vi "HandleError.vi"(8 "ErrorArray":errorcluster[](array[cluster])) -> (0 "ErrorArray":errorcluster[](array[cluster]), 4 "Stop":bool)   [LabVIEW 2014, in "TestBase.lvclass"]
uses:
  TestBase.lvclass
  Queue/clQueMsgType.ctl
  <vilib>/Utility/error.llb/Error Cluster From Error Code.vi
  <vilib>/ErrorRing/Error Ring.xnode
  <userlib>/NIST/NISTErrorLib/NISTErrorLib.lvlib
panel:
  out "XML_Out":string[](array[string])
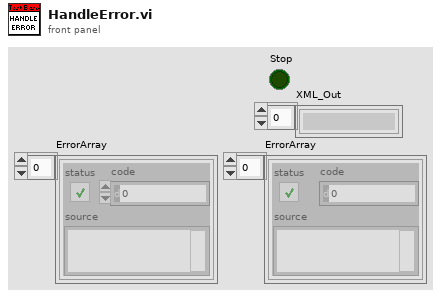
[diagram p1: front panel]
types:
  T1 = typedef "TestBase.lvclass/clQueMsgType.ctl" = cluster{"Message":string, "Data":variant}
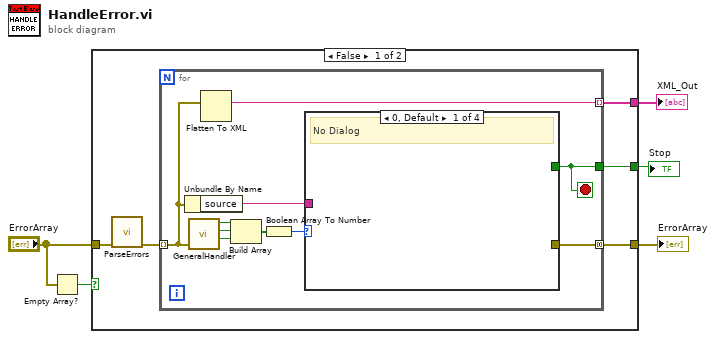
[diagram p0: block diagram]
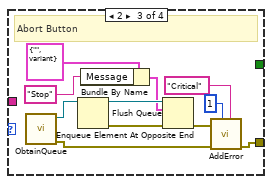
[diagram p4: hidden frame]
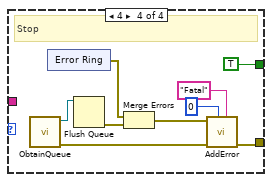
[diagram p5: hidden frame]
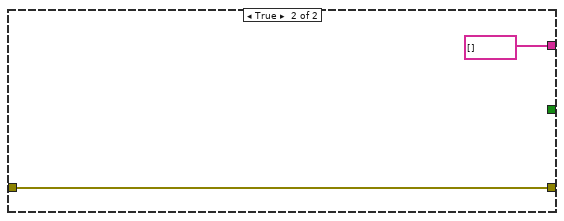
[diagram p6: hidden frame]
diagram:
  n1 = Empty Array?(array="ErrorArray") -> (empty?=w5:bool)
  n2 = case shown="False" w5 {
    tunnel: "ErrorArray" -> [w10 w48]
    tunnel: [w7 w48] -> w3
    tunnel: [w8 string[] [] ("XML_Out")] -> w2
    tunnel: [w6 _] -> w1
    frame False {
      n3 = call <userlib>:"ParseErrors.vi"("ErrorArray"=w10) -> ("ErrorArray"=w9:errorcluster[])  [unwired: 8 in, 2 out]
      n4 = for {
        tunnel: w9 -> [w20] mode=indexing
        tunnel: [w16] -> w8 mode=indexing
        tunnel: [w12] -> w7 mode=concatenating
        tunnel: [w11] -> w6
        stop <- w11 stop-if-true
        n5 = Unbundle By Name(w20) -> ("source"=w13:string)
        n6 = call <userlib>:"GeneralHandler.vi"("error in (no error)"=w20) -> ("Stop"=w17:bool, "Abort"=w18:bool, "Continue"=w19:bool)  [unwired: 7 in, 1 out]
        n7 = Flatten To XML(anything=w20) -> (xml string=w16:string)
        n8 = Build Array(w19, w18, w17) -> (w15:bool[])
        n9 = Boolean Array To Number(Boolean array=w15) -> (number=w14:u32)
        n10 = case shown="0, Default" w14 {
          tunnel: w13 -> [_ w21 _ _]
          tunnel: [_ _ w24 w40] -> w12
          tunnel: [_ _ _ TRUE] -> w11
          frame 0, Default {
            # "No Dialog"
          }
          frame 1 {
            # "Continue"
            n11 = case shown="\"Log\"" w21 {
              frame "False", Default {
              }
              frame "Log" {
                # "TODO: Add Logging"
              }
            }
          }
          frame 2 {
            # "Abort Button"
            n12 = call "ObtainQueue.vi"() -> ("ErrorArray."=w25:errorcluster[], "TstQue"=w32:refnum<queue>)  [unwired: 10 in]
            n13 = Flush Queue(queue=w32) -> (queue out=w28:refnum<queue>, error out=w31:errorcluster)  [unwired: 1 in, 1 out]
            n14 = Bundle By Name(cluster=T1 {"Message"="", "Data"=variant} ("clQueMsgType"), "Message"="Stop") -> (w27:T1)
            n15 = Enqueue Element At Opposite End(queue=w28, element=w27, error in (no error)=w31) -> (error out=w26:errorcluster)  [unwired: 1 in, 2 out]
            n16 = call <userlib>:"AddError.vi"("Severity"="Critical", "Priority"=u8 1, "ErrorArray"=w25, "error in (no error)"=w26) -> ("ErrorArray"=w24:errorcluster[])  [unwired: 6 in, 1 out]
          }
          frame 4 {
            # "Stop"
            n17 = call "ObtainQueue.vi"() -> ("ErrorArray."=w34:errorcluster[], "TstQue"=w41:refnum<queue>)  [unwired: 10 in]
            n18 = xnode "Error Ring"() -> ("error out"=w36:errorcluster)
            n19 = Flush Queue(queue=w41) -> (error out=w37:errorcluster)  [unwired: 1 in, 2 out]
            n20 = Merge Errors(w36, w37) -> (w35:errorcluster)
            n21 = call <userlib>:"AddError.vi"("Severity"="Fatal", "Priority"=u8 0, "ErrorArray"=w34, "error in (no error)"=w35) -> ("ErrorArray"=w40:errorcluster[])  [unwired: 6 in, 1 out]
          }
        }
      }
    }
    frame True {
    }
  }
  "ErrorArray" <- w3
  "Stop" <- w1
  "XML_Out" <- w2
